vi "Write DVR.vi"(8 "error in (no error)":errorcluster, 10 "DVR":refnum<data-value>, 11 "Data DVR Session in":refnum<class "Data DVR Session.lvclass">) -> (0 "error out":errorcluster, 3 "Data DVR Session out":refnum<class "Data DVR Session.lvclass">)   [LabVIEW 2014, in "Data DVR Session.lvclass"]
uses:
  Data DVR Session.lvclass
  Data/Data.lvclass
  Data DVR Session.lvclass/Data DVR Session.ctl
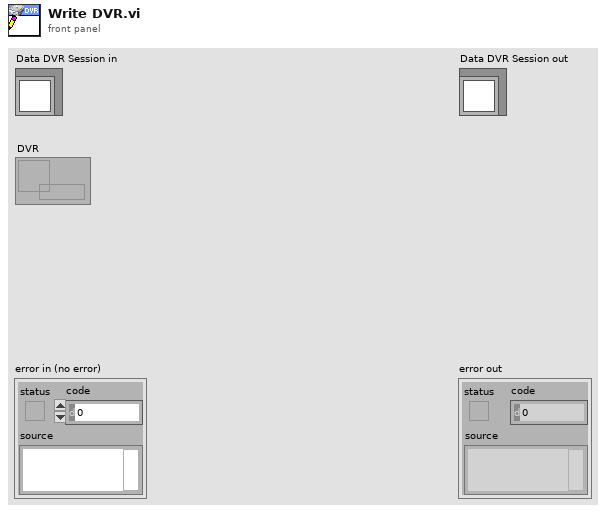
[diagram p1: front panel]
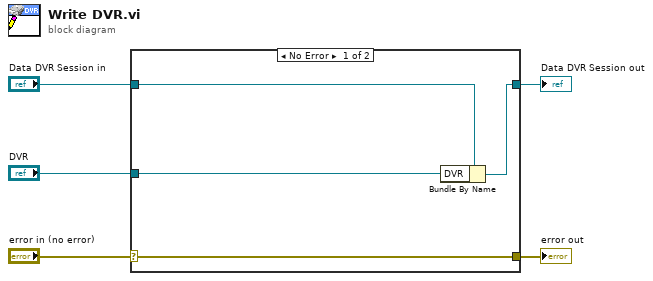
[diagram p0: block diagram]
diagram:
  n1 = case shown="No Error" "error in (no error)" {
    selector: "error in (no error)" -> [w9 w10]
    tunnel: [w9 w10] -> w4
    tunnel: [w7 w11] -> w2
    tunnel: "Data DVR Session in" -> [w8 w11]
    tunnel: "DVR" -> [w6 _]
    frame No Error {
      n2 = Bundle By Name(cluster=w8, "DVR"=w6) -> (w7:refnum<class "Data DVR Session.lvclass">)
    }
    frame Error {
    }
  }
  "error out" <- w4
  "Data DVR Session out" <- w2
